vi "Run All.vi"(8 "error in (no error)":errorcluster, 11 "Thread Manager in":refnum<class "Thread Manager.lvclass">) -> (0 "error out":errorcluster, 3 "Thread Manager out":refnum<class "Thread Manager.lvclass">)   [LabVIEW 2019, in "DSF Core.lvlib" / "Thread Manager.lvclass"]
uses:
  Thread Manager.lvclass
  Thread Manager.lvclass/Thread Manager.ctl
  Thread/Thread.lvclass
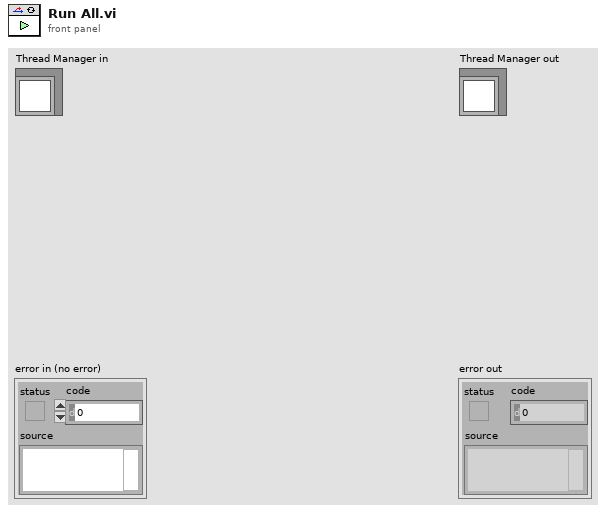
[diagram p1: front panel]
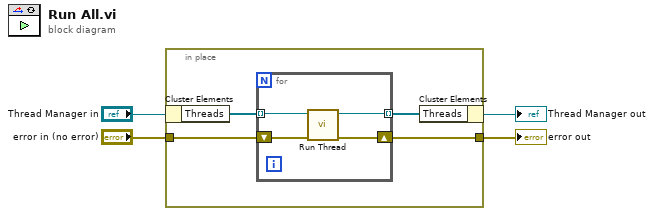
[diagram p0: block diagram]
diagram:
  n1 = in-place {
    in-place-border: [w6] -> w1
    in-place-border: "error in (no error)" -> [w5]
    n2 = in-place-cluster #1("Thread Manager in") -> ("Threads"=w8:refnum<class "Thread.lvclass">[])
    n3 = for {
      tunnel: w8 -> [w12] mode=indexing
      tunnel: [w11] -> w7 mode=indexing
      shift-right: [w10] -> w6
      shift-left: w5 -> [w9]
      n4 = call "Run Thread.vi"("error in (no error)"=w9, "Thread in"=w12) -> ("error out"=w10:errorcluster, "Thread out"=w11:refnum<class "Thread.lvclass">)  [unwired: 8 in]
    }
    n5 = in-place-cluster #1("Threads"=w7) -> (→"Thread Manager out":refnum<class "Thread Manager.lvclass">)
  }
  "error out" <- w1
